vi "test Launch Monitor.vi"(8 "error in (no error)":errorcluster, 11 "TestCase in":refnum<class "Monitor Test.lvclass">) -> (0 "error out":errorcluster, 3 "TestCase out":refnum<class "Monitor Test.lvclass">)   [LabVIEW 2017, in "Monitor Test.lvclass"]
uses:
  Monitor Test.lvclass
  Source/Monitor Data/Actor Data.ctl
  <vilib>/ActorFramework/Message Enqueuer/Message Enqueuer.lvclass
  Source/Monitored Actor/Monitored Actor/Monitored Actor.lvclass
  C:/Program Files (x86)/National Instruments/LabVIEW 2017/vi.lib/ActorFramework/Actor/Actor.lvclass
  <vilib>/ActorFramework/Message Enqueuer/Message Enqueuer.lvclass/Message Enqueuer.ctl
  <vilib>/ActorFramework/Message Enqueuer/Enqueue.vi
  <vilib>/ActorFramework/Stop Msg/Stop Msg.lvclass
  C:/Program Files (x86)/National Instruments/LabVIEW 2017/vi.lib/ActorFramework/Message/Message.lvclass
  <vilib>/ActorFramework/Message Priority Queue/Priority Enqueue.vi
  <vilib>/ActorFramework/Actor/Actor.lvclass
  Debug Monitor/Debug Monitor.lvclass
  Source/Monitor Data/Monitor Data.lvclass
panel:
  out "Actor Data":T1={"Actor Type"="", "Actor Cores"=[], "Self"=refnum, "Caller"=refnum, "Actor Label"="", "Last Ping"=-1.0}
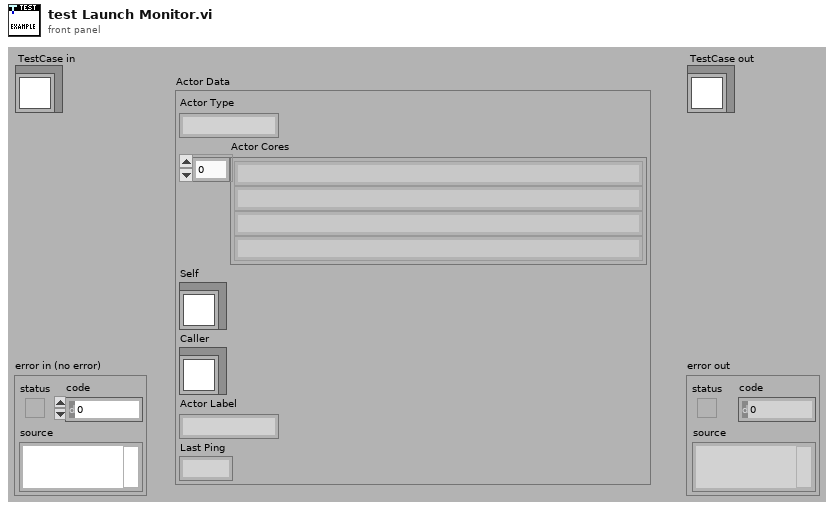
[diagram p1: front panel]
types:
  T1 = typedef "MGI-Monitored Actor Core.lvlib/Monitor Data.lvclass/Actor Data.ctl" = cluster{"Actor Type":string, "Actor Cores":string[], "Self":refnum<class "Message Enqueuer.lvclass">, "Caller":refnum<class "Message Enqueuer.lvclass">, "Actor Label":string, "Last Ping":dbl}
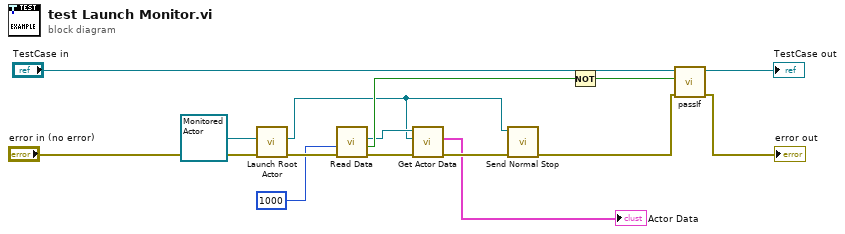
[diagram p0: block diagram]
diagram:
  n1 = call <vilib>:"Launch Root Actor.vi"("error in (no error)"="error in (no error)", "Actor"=refnum<class "Monitored Actor.lvclass"> refnum ("MGI-Monitored Actor Core.lvlib:Monitored Actor.lvclass")) -> ("error out"=w12:errorcluster, "Actor's Enqueuer"=w3:refnum<class "Message Enqueuer.lvclass">)  [unwired: 8 in]
  n2 = call "Read Data.vi"("error in (no error)"=w12, "timeout in ms (-1)"=1000) -> ("error out"=w4:errorcluster, "timed out?"=w10:bool, "Monitor Data"=w5:refnum<class "Monitor Data.lvclass">)  [unwired: 7 in]
  n3 = call "Get Actor Data.vi"("error in (no error)"=w4, "Actor's Self Q"=w3, "Monitor Data in"=w5) -> ("error out"=w2:errorcluster, "Actor Data"=→"Actor Data":T1)  [unwired: 5 in, 2 out]
  n4 = call <vilib>:"Send Normal Stop.vi"("error in (no error)"=w2, "Message Enqueuer"=w3) -> ("error out"=w9:errorcluster)  [unwired: 9 in]
  n5 = Not(x=w10) -> (.not. x?=w7:bool)
  n6 = call-dynamic "passIf.vi"("error in (no error)"=w9, "pass"=w7, "TestCase in"="TestCase in") -> ("error out"=→"error out":errorcluster, "TestCase out"=→"TestCase out":refnum<class "Monitor Test.lvclass">)  [unwired: 7 in]
